vi "replaceCategoryUpdateConditionToken.vi"(8 "error in (no error)":errorcluster, 10 "Query In":string, 11 "Credit Transaction in":refnum<class "CreditTransaction.lvclass">) -> (0 "error out":errorcluster, 2 "Query Out":string, 3 "Credit Transaction out":refnum<class "CreditTransaction.lvclass">)   [LabVIEW 2020]
uses:
  CreditTransaction.lvclass
  Transaction/Transaction.lvclass
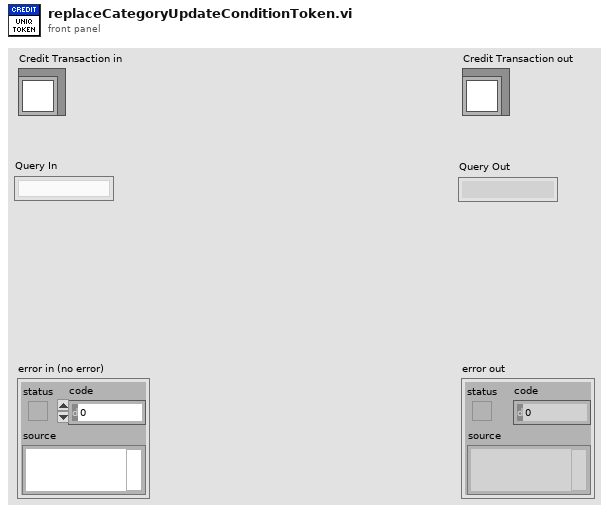
[diagram p1: front panel]
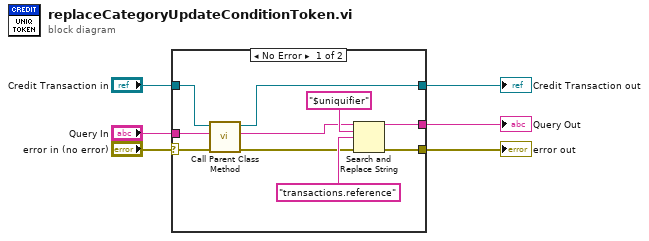
[diagram p0: block diagram]
diagram:
  n1 = case shown="No Error" "error in (no error)" {
    selector: "error in (no error)" -> [w10 w17]
    tunnel: "Query In" -> [w13 w18]
    tunnel: [w14 w18] -> w4
    tunnel: [w9 w17] -> w3
    tunnel: "Credit Transaction in" -> [w8 w19]
    tunnel: [w7 w19] -> w5
    frame No Error {
      n2 = call-parent "Call Parent Class Method"("error in (no error)"=w10, "Query In"=w13, "Transaction in"=w8) -> ("error out"=w11:errorcluster, "Query Out"=w12:string, "Transaction out"=w7:refnum<class "CreditTransaction.lvclass">)  [unwired: 6 in]
      n3 = Search and Replace String(input string=w12, search string="$uniquifier", replace string="transactions.reference", error in=w11) -> (result string=w14:string, error out=w9:errorcluster)  [unwired: 4 in, 2 out]
    }
    frame Error {
    }
  }
  "error out" <- w3
  "Credit Transaction out" <- w5
  "Query Out" <- w4
